vi "Wire Nodes Together.vi"(7 "Shift Pressed?":bool, 8 "error in (no error)":errorcluster, 11 "VI Ref":refnum<vi>) -> (0 "error out":errorcluster, 3 "dup VI":refnum<vi>)   [LabVIEW 2014]
doc: "Connects compatible terminals between multiple selected diagram objects. This shortcut will wire compatible data types between the objects in a left-to-right fashion. If [Shift] is also pressed, LabVIEW will perform a diagram cleanup of the selected objects after wiring them together.\n\nDefault Shortcut - [W]"
uses:
  <vilib>/Utility/traverseref.llb/TRef TravTarget.ctl
  <resource>/dialog/QuickDrop/plugins/_WireMultipleSupport/What to Wire.ctl
  <vilib>/Utility/traverseref.llb/VI Scripting - Traverse.lvlib
panel:
  in  "Undo Name":string="Wire Multiple Objects Together"
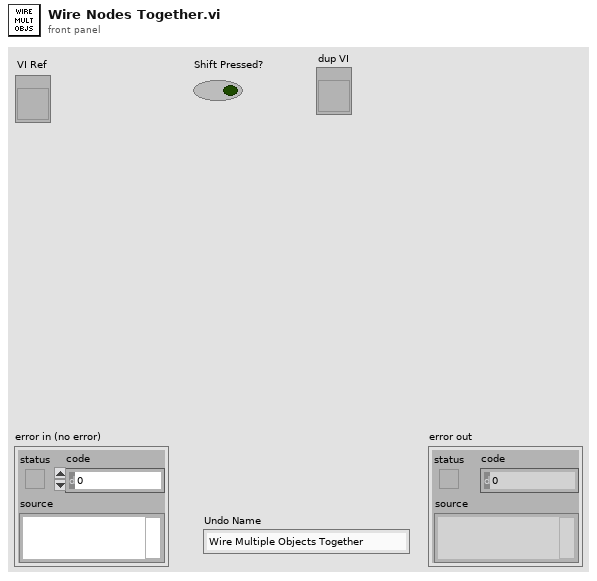
[diagram p1: front panel]
types:
  T1 = typedef "TRef TravTarget.ctl" = enum16{"FP", "BD", "Other"}
  T2 = typedef "What to Wire.ctl" = enum16{"node sinks", "node sources"}
  T3 = typedef "Node Terminal Info.ctl" = cluster{"Node Position (Left)":i32, "Node Ref":refnum<vi>, "Top Left":refnum<vi>, "Top Right":refnum<vi>, "Error Left":refnum<vi>, "Error Right":refnum<vi>}
  T4 = typedef "Available Non-Node.ctl" = cluster{"Left":i32, "Terminal":refnum<vi>}
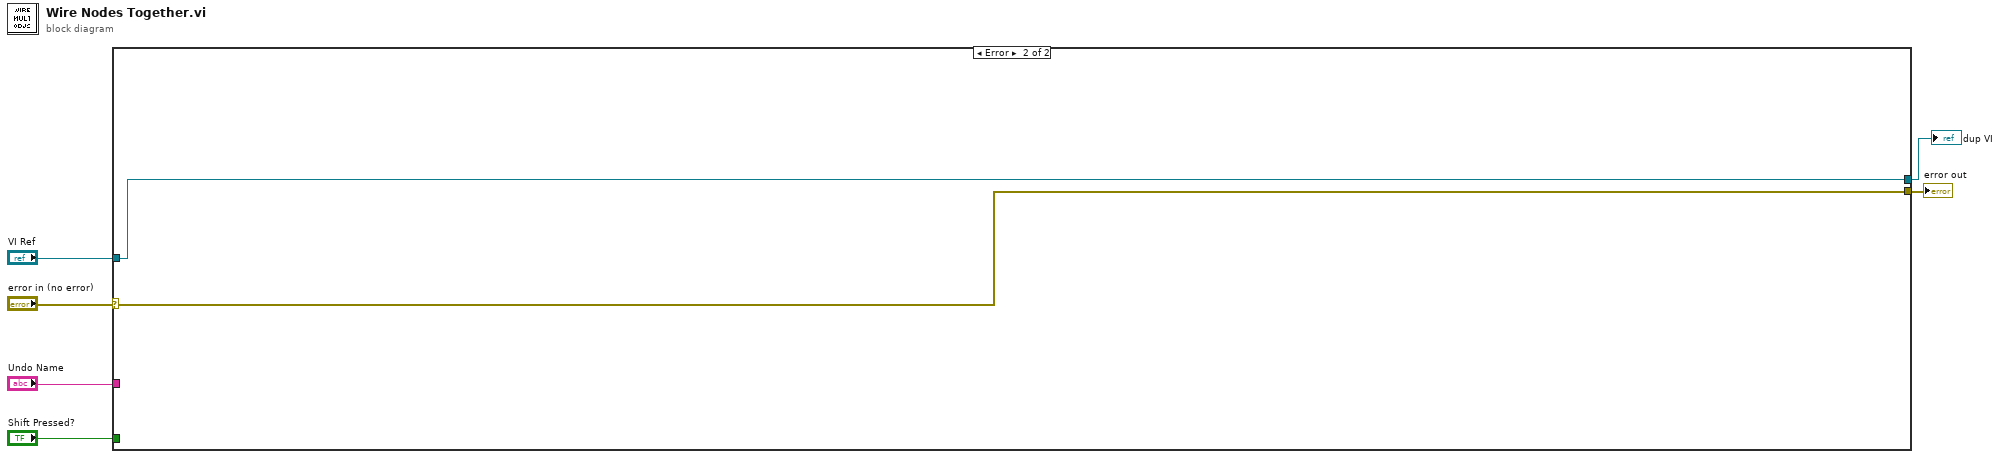
[diagram p0: block diagram]
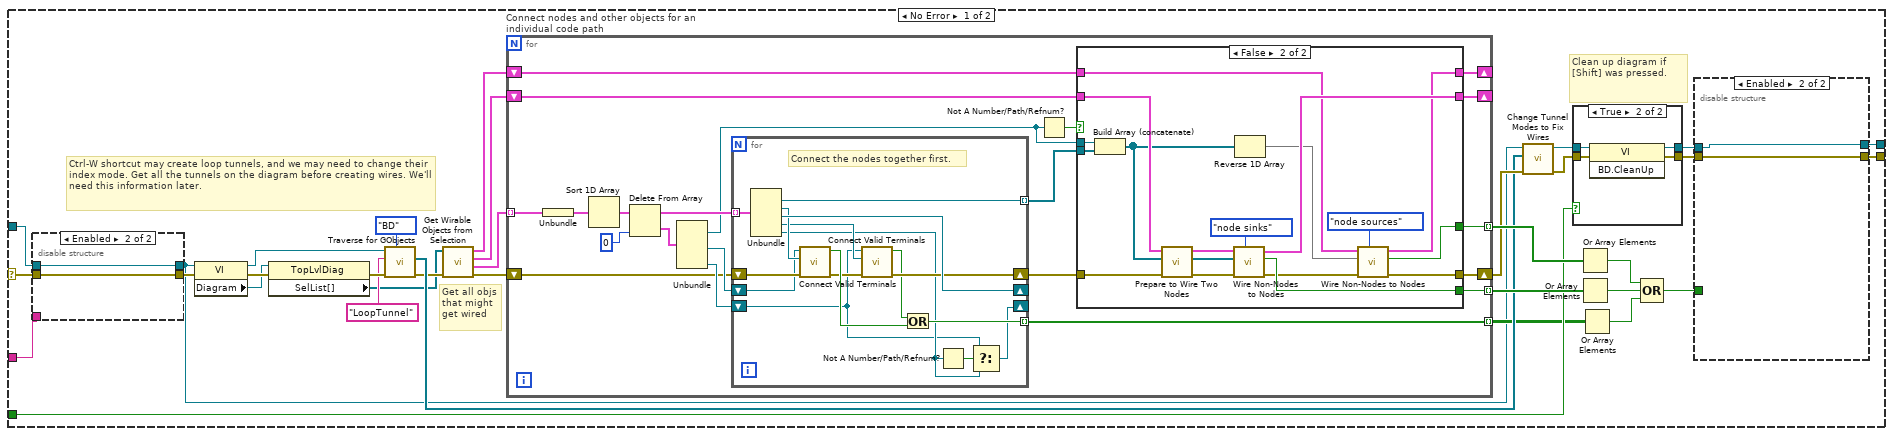
[diagram p2: hidden frame]
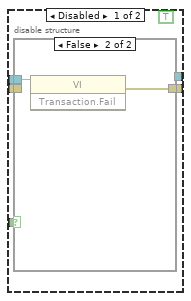
[diagram p3: hidden frame]
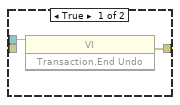
[diagram p4: hidden frame]
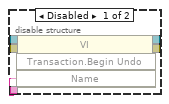
[diagram p5: hidden frame]
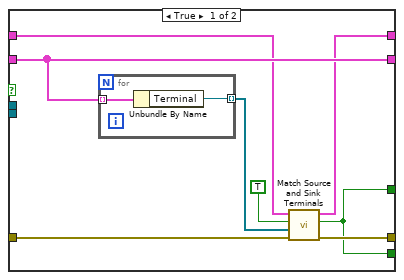
[diagram p6: hidden frame]
diagram:
  n1 = case shown="Error" "error in (no error)" {
    selector: "error in (no error)" -> [w39 w129]
    tunnel: [w35 w129] -> w5
    tunnel: "VI Ref" -> [w38 w128]
    tunnel: "Shift Pressed?" -> [w26 _]
    tunnel: "Undo Name" -> [w37 _]
    tunnel: [w7 w128] -> w1
    frame No Error {
      # "Get all objs\nthat might\nget wired"
      # "Ctrl-W shortcut may create loop tunnels, and we may need to change their index mode. Get all the tunnels on the diagram before creating wires. We'll need this information later."
      # "Clean up diagram if [Shift] was pressed."
      n2 = disable-structure shown="Enabled" {
        disable-tunnel: w39 -> [w54 w56]
        disable-tunnel: w38 -> [w53 w55]
        disable-tunnel: w37 -> [w52 _]
        disable-tunnel: [w51 w56] -> w36
        disable-tunnel: [w50 w55] -> w10
        frame Disabled {
          n3 = invoke class="VI" method="Transaction.Begin Undo"(reference=w53, error in=w54, "Name"=w52) -> (reference out=w50:refnum<vi>, error out=w51:errorcluster)  [unwired: 1 in, 2 out]
        }
        frame Enabled {
        }
      }
      n4 = property class="VI"(reference=w10, error in=w36) -> (reference out=w20:refnum<vi>, error out=w34:errorcluster, "Diagram"=w33:refnum<vi>)
      n5 = property class="TopLvlDiag"(reference=w33, error in=w34) -> (error out=w32:errorcluster, "SelList[]"=w13:refnum<vi>[])  [unwired: 1 out]
      n6 = call <vilib>:"Traverse for GObjects.vi"("Traverse Target"=TRef_TravTarget."BD", "error in (no error)"=w32, "Class Name"="LoopTunnel", "VI Refnum"=w20) -> ("error out"=w17:errorcluster, "References"=w18:refnum<vi>[])  [unwired: 4 in, 2 out]
      n7 = call <resource>:"Get Wirable Objects from Selection.vi"("error in (no error)"=w17, "SelList[]"=w13) -> ("error out"=w12:errorcluster, "Parsed Selection List (Geographic Rows)"=w11:cluster{"Selection List":T3[]}[], "Controls, Constants, and Source Tunnels"=w14:T4[], "Indicators and Sink Tunnels"=w15:T4[])  [unwired: 6 in]
      n8 = for "Connect nodes and other objects for an individual code path" {
        tunnel: [w77] -> w30 mode=indexing
        tunnel: [w76] -> w27 mode=indexing
        tunnel: [w72] -> w16 mode=indexing
        shift-right: [w75] -> w24
        shift-left: w12 -> [w62]
        shift-right: [w61] -> _
        shift-left: w15 -> [w68]
        shift-right: [w60] -> _
        shift-left: w14 -> [w64]
        tunnel: w11 -> [w59] mode=indexing
        n9 = Unbundle(w59) -> ("Selection List"=w58:T3[])
        n10 = Sort 1D Array(array=w58) -> (sorted array=w71:T3[])
        n11 = Delete From Array(array=w71, index=0) -> (deleted portion=w74:T3, array with subset deleted=w73:T3[])  [unwired: 1 in]
        n12 = Unbundle(w74) -> ("Node Ref"=w65:refnum<vi>, "Top Right"=w67:refnum<vi>, "Error Right"=w66:refnum<vi>)  [unwired: 3 out]
        n13 = for {
          shift-right: [w113] -> w70
          shift-left: w62 -> [w117]
          tunnel: w73 -> [w121] mode=indexing
          shift-right: [w118] -> _
          shift-left: w67 -> [w110]
          tunnel: [w119] -> w72 mode=indexing
          tunnel: [w120] -> w69 mode=indexing
          shift-right: [w106] -> _
          shift-left: w66 -> [w107]
          # "Connect the nodes together first."
          n14 = Unbundle(w121) -> ("Node Ref"=w120:refnum<vi>, "Top Left"=w115:refnum<vi>, "Top Right"=w118:refnum<vi>, "Error Left"=w112:refnum<vi>, "Error Right"=w108:refnum<vi>)  [unwired: 1 out]
          n15 = call <resource>:"Connect Valid Terminals.vi"("error in (no error)"=w117, "Sink Term"=w115, "Source Term"=w110) -> ("error out"=w114:errorcluster, "Connection Made?"=w116:bool)  [unwired: 7 in]
          n16 = call <resource>:"Connect Valid Terminals.vi"("error in (no error)"=w114, "Sink Term"=w112, "Source Term"=w107) -> ("error out"=w113:errorcluster, "Connection Made?"=w111:bool)  [unwired: 7 in]
          n17 = Or(x=w111, y=w116) -> (x .or. y?=w119:bool)
          n18 = Not A Number/Path/Refnum?(number/path/refnum=w108) -> (NaN/Path/Refnum?=w109:bool)
          n19 = Select(t=w107, s=w109, f=w108) -> (s? t:f=w106:refnum<vi>)
        }
        n20 = Not A Number/Path/Refnum?(number/path/refnum=w65) -> (NaN/Path/Refnum?=w63:bool)
        n21 = case shown="False" w63 {
          tunnel: w70 -> [w84 w94]
          tunnel: w69 -> [_ w92]
          tunnel: [w78 w103] -> w77
          tunnel: [w78 w95] -> w76
          tunnel: w68 -> [w82 w97]
          tunnel: [w83 w100] -> w75
          tunnel: w65 -> [_ w105]
          tunnel: w64 -> [w85 w91]
          tunnel: [w81 w96] -> w61
          tunnel: [w85 w104] -> w60
          frame True {
            n22 = for {
              tunnel: w85 -> [w87] mode=indexing
              tunnel: [w86] -> w80 mode=indexing
              n23 = Unbundle By Name(w87) -> ("Terminal"=w86:refnum<vi>)
            }
            n24 = call <resource>:"Match Source and Sink Terminals.vi"("error in (no error)"=w84, "Node Terminals"=w80, "Node Sources?"=TRUE, "Available Non-Nodes in"=w82) -> ("error out"=w83:errorcluster, "Any Changes?"=w78:bool, "Available Non-Nodes out"=w81:T4[])  [unwired: 5 in]
          }
          frame False {
            n25 = Build Array (concatenate)(w105, w92) -> (w89:refnum<vi>[])
            n26 = call <resource>:"Prepare to Wire Two Nodes.vi"("error in (no error)"=w94, "Nodes"=w89, "Available Non-Nodes in"=w91) -> ("error out"=w93:errorcluster, "dup Nodes"=w88:refnum<vi>[], "Available Non-Nodes out"=w90:T4[])  [unwired: 6 in]
            n27 = call <resource>:"Wire Non-Nodes to Nodes.vi"("What to Wire"=What_to_Wire."node sinks", "error in (no error)"=w93, "Nodes"=w88, "Available Non-Nodes in"=w90) -> ("error out"=w101:errorcluster, "Any Changes?"=w103:bool, "Available Non-Nodes out"=w104:T4[])  [unwired: 5 in]
            n28 = Reverse 1D Array(array=w89) -> (reversed array=w98:refnum<vi>[])
            n29 = call <resource>:"Wire Non-Nodes to Nodes.vi"("What to Wire"=What_to_Wire."node sources", "error in (no error)"=w101, "Nodes"=w98, "Available Non-Nodes in"=w97) -> ("error out"=w100:errorcluster, "Any Changes?"=w95:bool, "Available Non-Nodes out"=w96:T4[])  [unwired: 5 in]
          }
        }
      }
      n30 = call <resource>:"Change Tunnel Modes to Fix Wires.vi"("error in (no error)"=w24, "All Tunnels (before wiring)"=w18, "VI"=w10) -> ("error out"=w23:errorcluster, "dup VI"=w9:refnum<vi>)  [unwired: 7 in]
      n31 = case shown="True" w26 {
        tunnel: w23 -> [w123 w127]
        tunnel: [w123 w126] -> w8
        tunnel: w9 -> [w122 w125]
        tunnel: [w122 w124] -> w25
        frame False {
        }
        frame True {
          n32 = invoke class="VI" method="BD.CleanUp"(reference=w125, error in=w127) -> (reference out=w124:refnum<vi>, error out=w126:errorcluster)  [unwired: 1 in, 1 out]
        }
      }
      n33 = Or Array Elements(Boolean array=w27) -> (logical OR=w28:bool)
      n34 = Or Array Elements(Boolean array=w30) -> (logical OR=w29:bool)
      n35 = Or Array Elements(Boolean array=w16) -> (logical OR=w19:bool)
      n36 = Compound Arithmetic op=OR(w28, w29, w19) -> (w31:bool)
      n37 = disable-structure shown="Enabled" {
        disable-tunnel: [w43 w49] -> w35
        disable-tunnel: w31 -> [w42 _]
        disable-tunnel: w25 -> [w41 w48]
        disable-tunnel: w8 -> [w40 w49]
        disable-tunnel: [_ w48] -> w7
        frame Disabled {
          (unwired) TRUE
          n38 = case shown="False" w42 {
            tunnel: w41 -> [w44 w46]
            tunnel: [w45 w47] -> w43
            tunnel: w40 -> [_ _]
            frame True {
              n39 = invoke class="VI" method="Transaction.End Undo"(reference=w44) -> (error out=w45:errorcluster)  [unwired: 2 in, 2 out]
            }
            frame False {
              n40 = invoke class="VI" method="Transaction.Fail"(reference=w46) -> (error out=w47:errorcluster)  [unwired: 2 in, 2 out]
            }
          }
        }
        frame Enabled {
        }
      }
    }
    frame Error {
    }
  }
  "error out" <- w5
  "dup VI" <- w1
